vi "DRIVE_STRAIGHT_PE.vi"(10 "argv":string[](array[string]), 11 "args":u8) -> ()   [LabVIEW 2014]
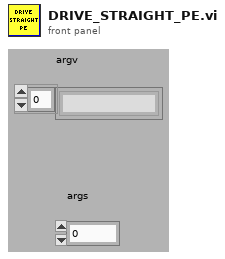
[diagram p1: front panel]
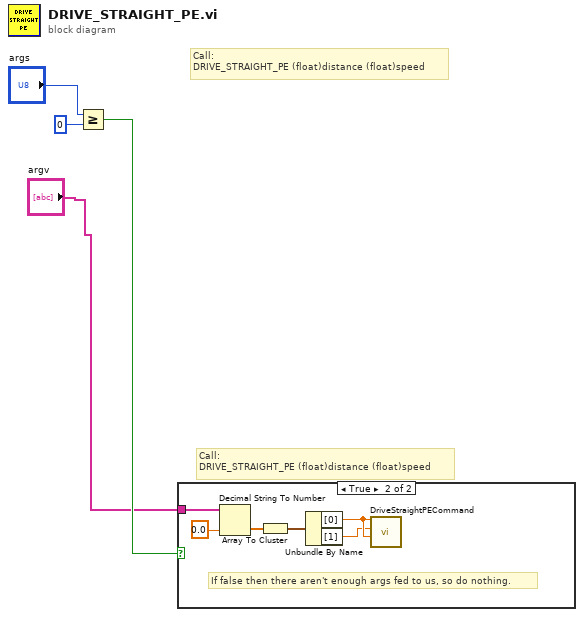
[diagram p0: block diagram]
diagram:
  # "Call:\nDRIVE_STRAIGHT_PE (float)distance (float)speed"
  # "Call:\nDRIVE_STRAIGHT_PE (float)distance (float)speed"
  n1 = Greater Or Equal?(x="args", y=u8 0) -> (x >= y?=w4:bool)
  n2 = case shown="True" w4 {
    tunnel: "argv" -> [_ w10]
    frame False {
    }
    frame True {
      # "If false then there aren't enough args fed to us, so do nothing."
      n3 = Decimal String To Number(string=w10, default (0L)=0.0 ("default (0 I32)")) -> (number=w8:dbl[])  [unwired: 2 out]
      n4 = Array To Cluster(array=w8) -> (cluster=w7:cluster{"[0]":dbl, "[1]":dbl})
      n5 = Unbundle By Name(w7) -> ("[0]"=w6:dbl, "[1]"=w5:dbl)
      n6 = call "DriveStraightPECommand.vi"("Fwd Bwd"=w6, "Delay ms"=w5, "distance"=w6) -> ()  [unwired: 9 in]
    }
  }
